vi "실습 9-4 2진 파일에 쓰기.vi"() -> ()   [LabVIEW 2014]
uses:
  <vilib>/Analysis/NI_AALBase.lvlib
panel:
  out "웨이브폼 그래프":dbl[][](graph)
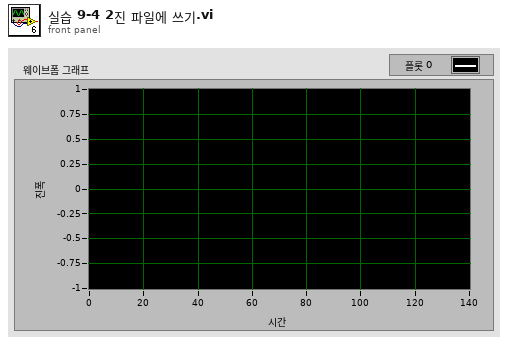
[diagram p1: front panel]
types:
  T1 = enum16{"big-endian, network order", "native, host order", "little-endian"}
  T2 = enum16{"open", "replace", "create", "open or create", "replace or create", "replace or create with confirmation"}
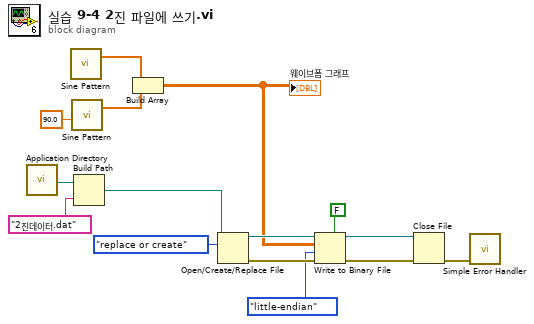
[diagram p0: block diagram]
diagram:
  n1 = call <vilib>:"Application Directory.vi"() -> ("Application Directory"=w4:path)
  n2 = call <vilib>:"Sine Pattern.vi"() -> ("Sinusoidal Pattern"=w8:dbl[])  [unwired: 4 in, 1 out]
  n3 = call <vilib>:"Sine Pattern.vi"("phase(degrees)"=90.0) -> ("Sinusoidal Pattern"=w7:dbl[])  [unwired: 3 in, 1 out]
  n4 = Build Path(base path=w4, name or relative path="2진데이터.dat" ("이름 또는 상대 경로")) -> (appended path=w2:path)
  n5 = Build Array(w8, w7) -> (w6:dbl[][])
  "웨이브폼 그래프" <- w6
  n6 = Open/Create/Replace File(file path (use dialog)=w2, operation (0:open)=T2."replace or create" ("동작(0:open)")) -> (refnum out=w14:refnum<file>, error out=w12:errorcluster)  [unwired: 4 in, 1 out]
  n7 = Write to Binary File(file (use dialog)=w14, data=w6, error in=w12, 5:FALSE ("배열 또는 문자열 크기를 앞에 추가? (참)"), 9:T1."little-endian" ("바이트 순서(0:big-endian, network order)")) -> (refnum out=w13:refnum<file>, error out=w11:errorcluster)  [unwired: 1 in, 1 out]
  n8 = Close File(refnum=w13, error in=w11) -> (error out=w1:errorcluster)  [unwired: 1 out]
  n9 = call <vilib>:"Simple Error Handler.vi"("error in (no error)"=w1) -> ()  [unwired: 4 in, 5 out]
